vi "statistics.vi"() -> ()   [LabVIEW 2025]
uses:
  <vilib>/regexp/Match Regular Expression.xnode
panel:
  in  "path":path=path "/git/portfolio/jobPortal2/testerOprogramowania/backup"
  out "xy graph":cluster{"X":dbl, "Y":dbl}[](graph)
  out "error out":errorcluster
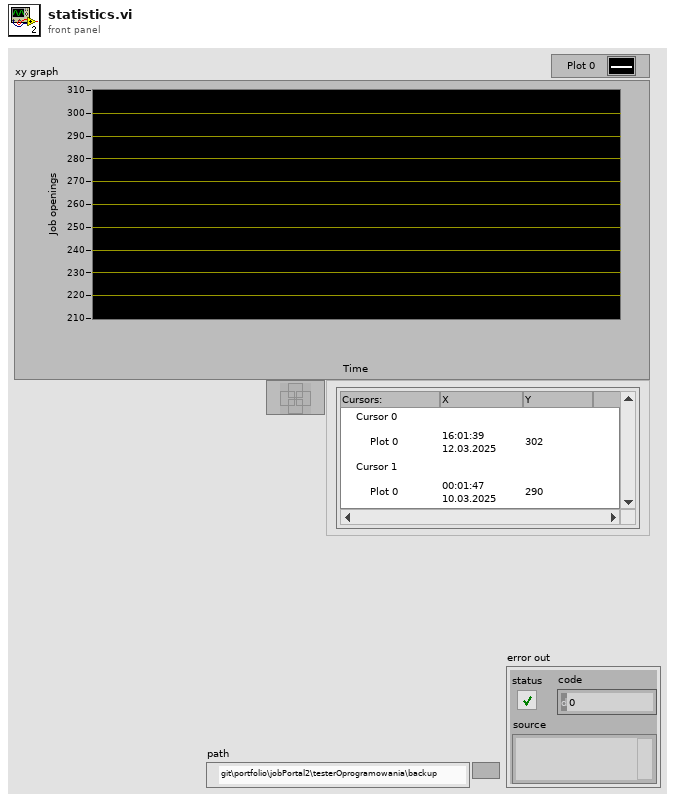
[diagram p1: front panel]
types:
  T1 = cluster{"index":i32, "title":string, "link":string, "salary":string, "employer":string, "employerLink":string, "level":string, "workplace":string, "keywords":string, "userNote":string, "userNote2":string, "userNote3":string, "userNote4":string, "userNote5":string}[]
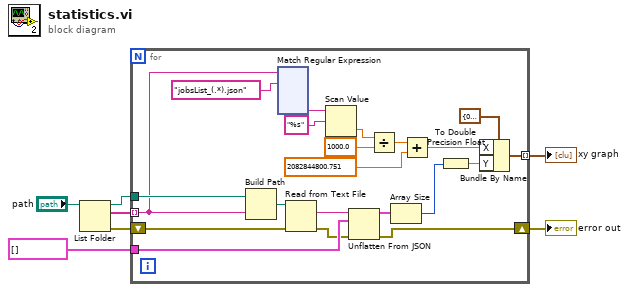
[diagram p0: block diagram]
diagram:
  n1 = List Folder(path="path") -> (path out=w5:path, filenames=w6:string[], error out=w4:errorcluster)  [unwired: 3 in, 1 out]
  n2 = for {
    tunnel: T1 [] -> [w28]
    tunnel: w6 -> [w12] mode=indexing
    tunnel: w5 -> [w24]
    shift-right: [w21] -> w3
    shift-left: w4 -> [w23]
    tunnel: [w14] -> w1 mode=indexing
    n3 = Build Path(base path=w24, name or relative path=w12) -> (appended path=w25:path)
    n4 = xnode "Match Regular Expression"("input string"=w12, "regular expression"="jobsList_(.*).json") -> ("submatch 1"=w8:string)  [unwired: 4 in, 5 out]
    n5 = Read from Text File(file (use dialog)=w25, error in=w23) -> (text=w27:string, error out=w22:errorcluster)  [unwired: 2 in, 2 out]
    n6 = Scan Value(string=w8, format string="%s") -> (value=w20:dbl)  [unwired: 1 in, 1 out]
    n7 = Unflatten From JSON(JSON string=w27, type and defaults=w28, error in (no error)=w22) -> (value=w26:T1, error out=w21:errorcluster)  [unwired: 4 in]
    n8 = Divide(x=w20, y=1000.0) -> (x/y=w17:dbl)
    n9 = Array Size(array=w26) -> (size(s)=w10:i32)
    n10 = Add(x=w17, y=2082844800.751 ("x-y")) -> (x+y=w15:dbl)
    n11 = To Double Precision Float(number=w10) -> (double precision float=w9:dbl)
    n12 = Bundle By Name(cluster=cluster{"X":dbl, "Y":dbl} {"X"=0.0, "Y"=0.0}, "X"=w15, "Y"=w9) -> (w14:cluster{"X":dbl, "Y":dbl})
  }
  "error out" <- w3
  "xy graph" <- w1
